vi "File_HandleSegmentation.vi"(8 "error in (no error)":errorcluster, 9 "Segment by":T1=enum."Size (MB)", 10 "Segment Every":dbl, 11 "File in":refnum<class "File.lvclass">) -> (0 "error out":errorcluster, 1 "old path":path, 2 "Segment?":bool, 3 "File out":refnum<class "File.lvclass">)   [LabVIEW 2024, in "File.lvclass"]
doc: "Determine whether the segmentation conditions are met and if so, close the file and start a new TDMS file to log to (i.e. segment)."
uses:
  File.lvclass
  SegmentationOptions.ctl
  File.lvclass/File.ctl
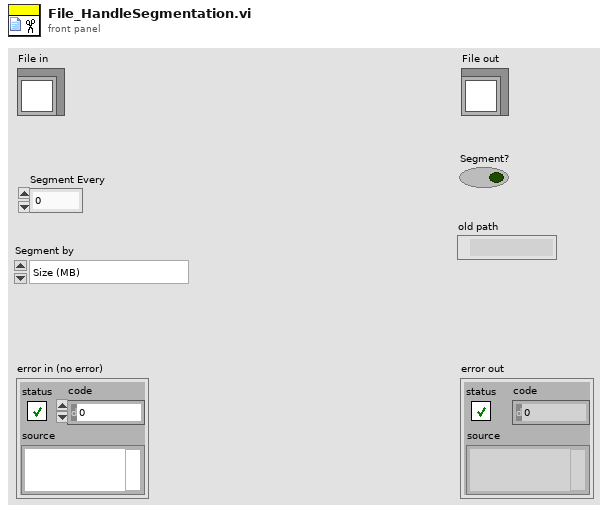
[diagram p1: front panel]
types:
  T1 = typedef "SegmentationOptions.ctl" = enum16{"Time (s)", "Size (MB)"}
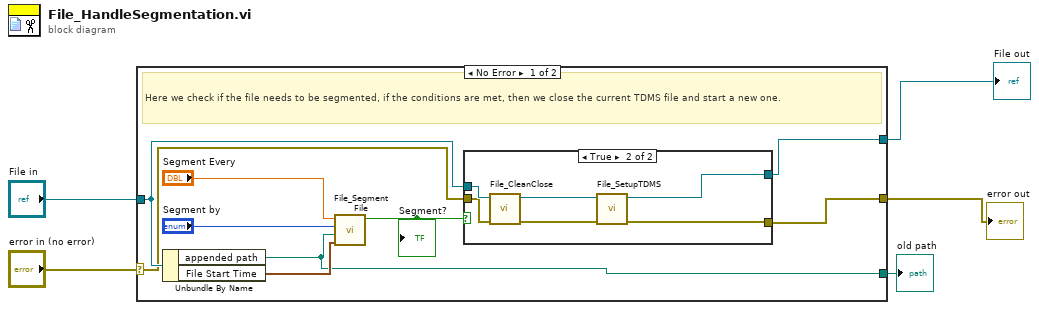
[diagram p0: block diagram]
diagram:
  n1 = case shown="No Error" "error in (no error)" {
    selector: "error in (no error)" -> [w10 w24]
    tunnel: [w11 w24] -> w4
    tunnel: [w12 w23] -> w2
    tunnel: "File in" -> [w13 w23]
    tunnel: [w6 _] -> w1
    frame No Error {
      # "Here we check if the file needs to be segmented, if the conditions are met, then we close the current TDMS file and start a new one."
      n2 = Unbundle By Name(w13) -> ("appended path"=w6:path, "File Start Time"=w7:timestamp)
      n3 = call "File_Segment File.vi"("current time in"=w7, "path in"=w6, "Segment by"="Segment by", "Segment Every"="Segment Every") -> ("Boolean"=w14:bool)  [unwired: 7 in]
      "Segment?" <- w14
      n4 = case shown="True" w14 {
        tunnel: w10 -> [w15 w21]
        tunnel: w13 -> [w16 w22]
        tunnel: [w16 w18] -> w12
        tunnel: [w15 w17] -> w11
        frame False {
        }
        frame True {
          n5 = call-dynamic "File_CleanClose.vi"("error in (no error)"=w21, "File in"=w22) -> ("error out"=w19:errorcluster, "File out"=w20:refnum<class "File.lvclass">)  [unwired: 8 in]
          n6 = call-dynamic "File_SetupTDMS.vi"("error in (no error)"=w19, "File in"=w20) -> ("error out"=w17:errorcluster, "File out"=w18:refnum<class "File.lvclass">)  [unwired: 8 in]
        }
      }
    }
    frame Error {
    }
  }
  "error out" <- w4
  "File out" <- w2
  "old path" <- w1
